vi "write_to_db.vi"(0 "reference in":refnum<class "DA.lvclass">, 11 "error in (no error)":errorcluster) -> (4 "reference out":refnum<class "DA.lvclass">, 15 "error out":errorcluster)   [LabVIEW 2019, in "DA.lvclass"]
uses:
  DA.lvclass
  Logger_class/EventData.ctl
  Logger_class/Logger.lvclass
  Proccess_class/Proccess.lvclass
  D:/GIT H4000/H4000/src/Proccess_class/Proccess.lvclass
  Logger_class/EventType.ctl
  TypeDef/AlarmType.ctl
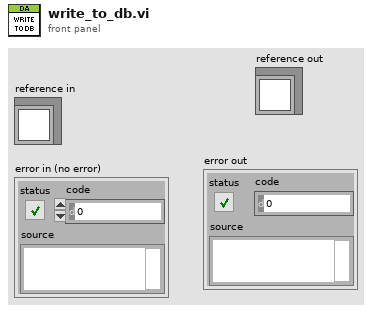
[diagram p1: front panel]
types:
  T1 = typedef "AlarmType.ctl" = enum16{"Normal", "Warning", "Alarm"}
  T2 = typedef "Logger.lvclass/EventType.ctl" = enum16{"DI", "DO", "DA", "AI", "AO", "AA", "CMD", "ERR", "ST"}
  T3 = typedef "Logger.lvclass/EventData.ctl" = cluster{"obj_tag":string, "event_tag":string, "Description":string, "EVENT TYPE":T4, "ALARM TYPE":T1, "Value DBL":dbl, "Value INT":i32, "Value STR":string, "Time Stamp":timestamp}
  T4 = typedef "Logger.lvclass/EventType.ctl" = enum16{"DI_LO", "DI_HI", "DO_LO", "DO_HI", "DA_LO", "DA_HI", "AA_LO", "AA_HI", "CMD", "ERR", "ST"}
  T5 = typedef "Proccess.lvclass/TAGs.ctl" = cluster{"TAG":string, "PTAG":string, "DESC":string}
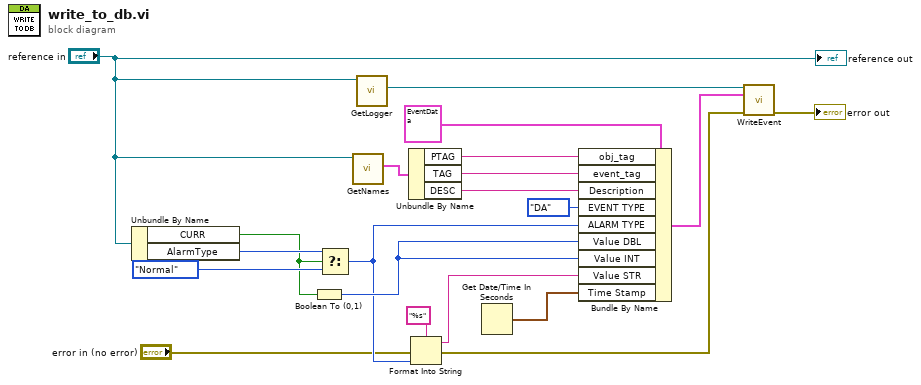
[diagram p0: block diagram]
diagram:
  n1 = Unbundle By Name("reference in") -> ("CURR"=w9:bool, "AlarmType"=w10:T1)
  n2 = Boolean To (0,1)(Boolean=w9) -> (0, 1=w8:i16)
  n3 = Select(t=w10, s=w9, f=AlarmType."Normal" ("ALARM TYPE")) -> (s? t:f=w5:T1)
  n4 = call "GetNames.vi"("Proccess in"="reference in") -> ("Tags"=w17:T5)  [unwired: 10 in]
  n5 = call "GetLogger.vi"("Proccess in"="reference in") -> ("Logger"=w19:refnum<class "Logger.lvclass">)  [unwired: 10 in]
  n6 = Unbundle By Name(w17) -> ("PTAG"=w15:string, "TAG"=w14:string, "DESC"=w13:string)
  n7 = Format Into String(format string="%s", error in="error in (no error)", w5) -> (resulting string=w4:string, error out=w2:errorcluster)  [unwired: 1 in]
  n8 = Get Date/Time In Seconds() -> (seconds since 1Jan1904=w7:timestamp)
  n9 = Bundle By Name(cluster=T3 {"obj_tag"="", "event_tag"="", "Description"="", "EVENT TYPE"=enum."DA_LO", "ALARM TYPE"=enum."Alarm", "Value DBL"=0.0, "Value INT"=0, "Value STR"="", "Time Stamp"=timestamp(0 s since 1904-01-01)} ("Event"), "obj_tag"=w15, "event_tag"=w14, "Description"=w13, "EVENT TYPE"=EventType."DA", "ALARM TYPE"=w5, "Value DBL"=w8, "Value INT"=w8, "Value STR"=w4, "Time Stamp"=w7) -> (w1:T3)
  n10 = call "WriteEvent.vi"("reference in"=w19, "Event"=w1, "error in (no error)"=w2) -> ("error out"=→"error out":errorcluster)  [unwired: 11 in, 1 out]
  "reference out" <- "reference in"
